vi "PythonIDE 3.vi"(7 "Python version":string="3.9", 9 "Processor":u16(ring) items=["SPIKE", "Pi"], 11 "Port":string) -> ()   [LabVIEW 2020]
uses:
  <vilib>/event_ctls.llb/eventvkey.ctl
  Serial_Global.vi
panel:
  out "Shift":bool
  in  "Explorer":u16(ring) items=["Explore...", "", "Arm", "Motors", "Scope", "Twin"]
  out "Buffer":i32(slide) scale=0.0..10000.0
  in  "Folder Path":path
  in  "Open PC":bool
  in  "reconnect":bool
  out "VKey":T1
  in  "Browser":bool
  in  "Tree":string(tree)
  in  "Spaces":bool
  in  "Name":string="main.py"
  in  "Save SPIKE":bool
  out "Script":string
  in  "Python Code":string
  out "Console":string
  in  "Clear":bool
  in  "Text.Font:Size":u32=12
  in  "Save Log":bool
  in  "Save PC":bool
  in  "stop":bool
  in  "Ctrl C":bool
  in  "run":bool
  # "PyVIEW IDE\nversion 0.1b10"
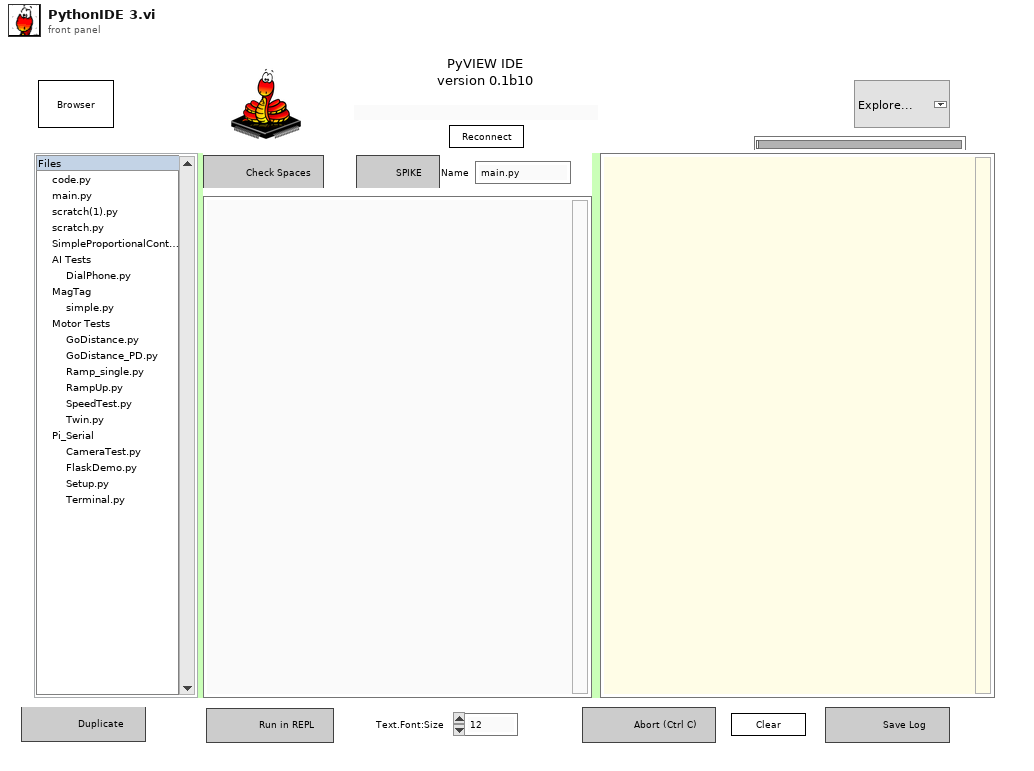
[diagram p1: front panel]
types:
  T1 = typedef "eventvkey.ctl" = enum16{"ASCII", "Enter", "Return", "Shift", "Ctrl", "Alt", "Cmd", "Opt", "Caps", "NumLock", "Clear", "Break", "Up", "Down", "Left", "Right", "Insert", "Delete", "Home", "End", "PageUp", "PageDown", "Escape", "Help", "Pause", "ScrollLock", "F1", "F2", "F3", "F4", "F5", "F6", "F7", "F8", "F9", "F10", "F11", "F12", "F13", "F14", "F15", "F16", "F17", "F18", "F19", "F20", "F21", "F22", "F23", "F24", "Play", "VolumeUp", "VolumeDown", "Mute", "Two Byte Char"}
  T2 = typedef "PythonCtrl.ctl" = cluster{"session":refnum<k35>, "PyPath":path, "Processor":enum16{"SPIKE", "Pi"}}
  T3 = enum8{"Enabled", "Disabled", "Disabled and Grayed Out"}
  T4 = typedef "Preferences.ctl" = cluster{"python":string, "arduino15":path, "arduino Lib":path, "pythonCode":path, "FontSize":u8}
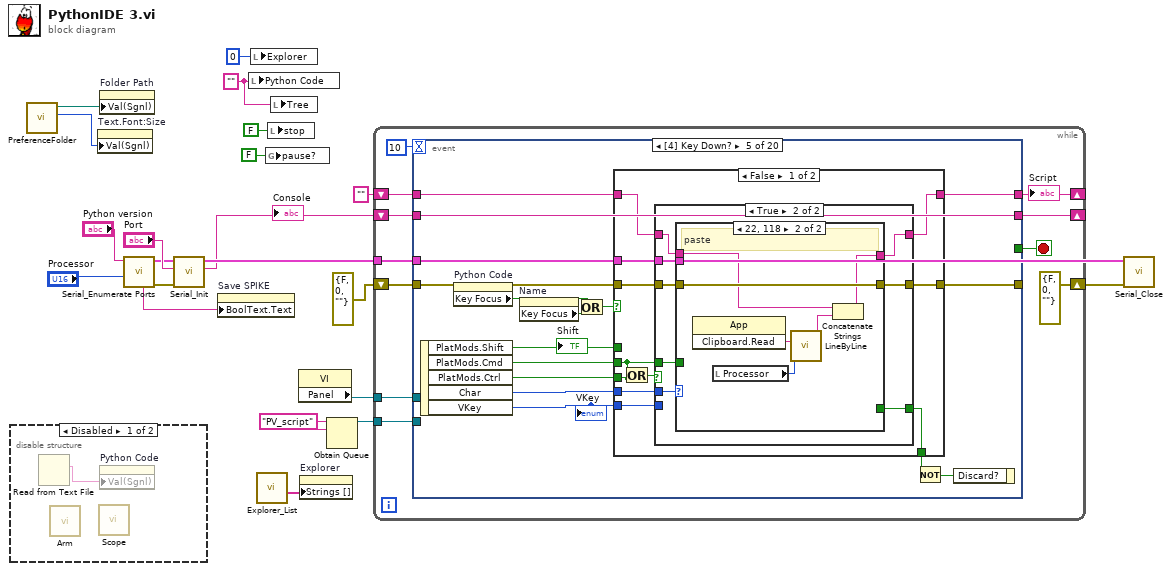
[diagram p0: block diagram]
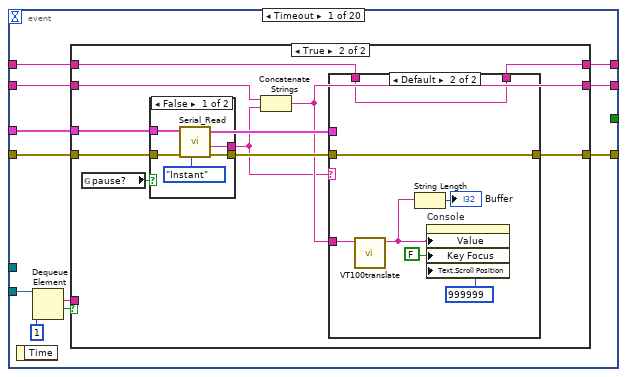
[diagram p2: hidden frame]
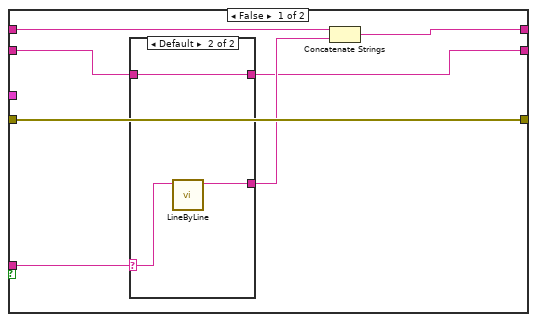
[diagram p3: hidden frame]
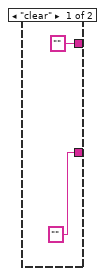
[diagram p4: hidden frame]
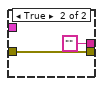
[diagram p5: hidden frame]
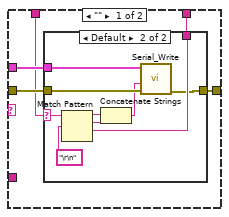
[diagram p6: hidden frame]
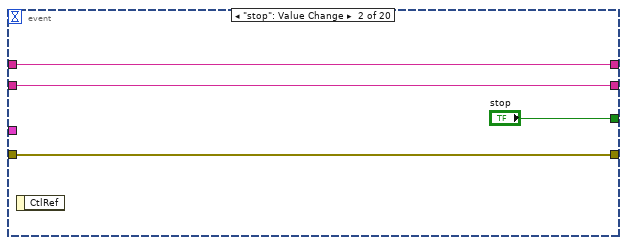
[diagram p8: hidden frame]
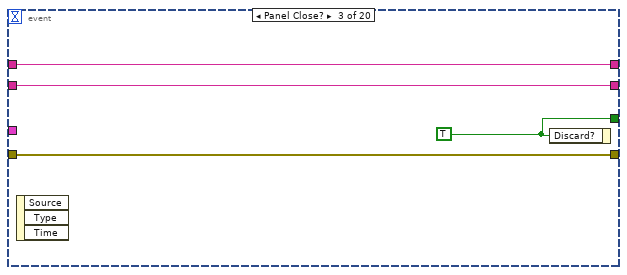
[diagram p9: hidden frame]
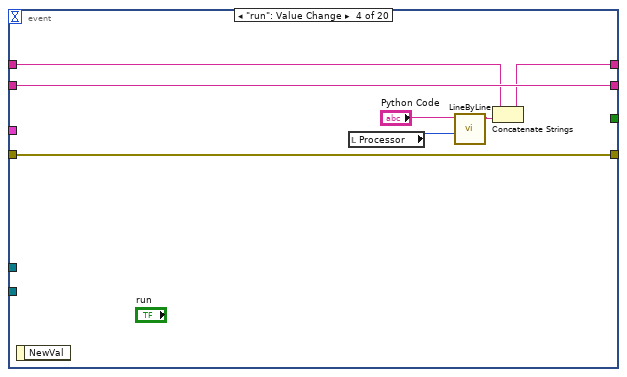
[diagram p10: hidden frame]
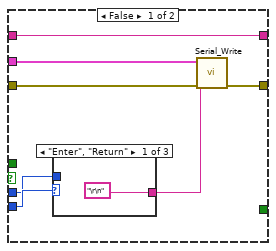
[diagram p11: hidden frame]
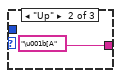
[diagram p12: hidden frame]
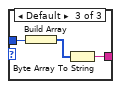
[diagram p13: hidden frame]
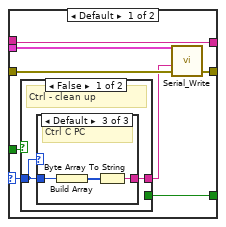
[diagram p14: hidden frame]
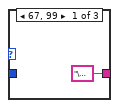
[diagram p15: hidden frame]
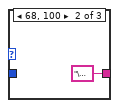
[diagram p16: hidden frame]
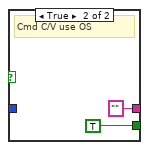
[diagram p17: hidden frame]
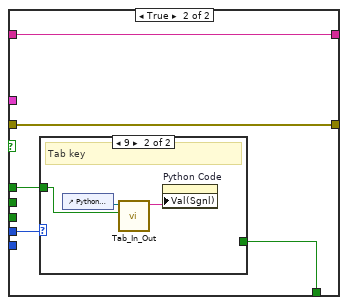
[diagram p18: hidden frame]
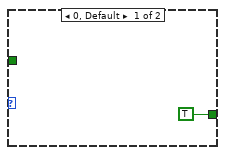
[diagram p19: hidden frame]
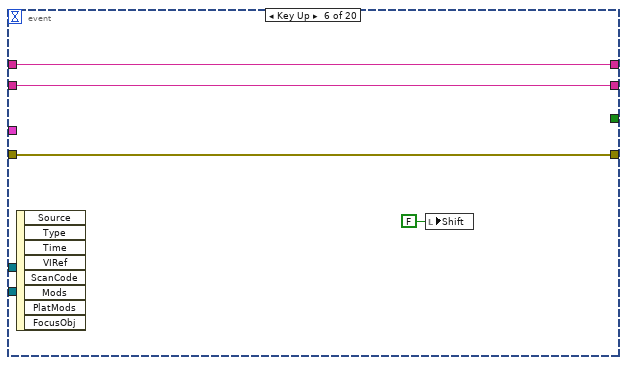
[diagram p20: hidden frame]
diagram:
  w6 = "PV_script" ("name (unnamed)")
  w11 = "" ("Python Code")
  n1 = disable-structure shown="Disabled" {
    frame Disabled {
      n2 = Read from Text File() -> (text=w22:string)  [unwired: 4 in, 3 out]
      n3 = call "Arm.vi"() -> ()  [unwired: 12 in]
      n4 = call "Scope.vi"() -> ()  [unwired: 12 in]
      n5 = property on="Python Code" class="Str"("Val(Sgnl)"=w22) -> ()  [unwired: 2 in, 2 out]
    }
    frame Enabled {
    }
  }
  n6 = call "PreferenceFolder.vi"() -> ("FontSize"=w9:u8, "pythonCode"=w10:path)  [unwired: 9 in, 1 out]
  n7 = property on="Text.Font:Size" class="DigNum (strict)"("Val(Sgnl)"=w9) -> ()  [unwired: 2 in, 2 out]
  n8 = property on="Folder Path" class="Path"("Val(Sgnl)"=w10) -> ()  [unwired: 2 in, 2 out]
  n9 = call "Serial_Enumerate Ports.vi"("Processor"="Processor", "Python version"="Python version") -> ("error out"=w15:errorcluster, "Python"=w17:T2, "name"=w1:string)  [unwired: 5 in, 2 out]
  n10 = call "Serial_Init.vi"("error in (no error)"=w15, "Port"="Port", "Python"=w17) -> ("Console"=w14:string, "Python out"=w16:T2)  [unwired: 6 in, 1 out]
  "Console" <- w14
  n11 = property on="Save SPIKE" class="Bool"("BoolText.Text"=w1) -> ()  [unwired: 2 in, 2 out]
  n12 = local write "Python Code"(w11) -> ()
  n13 = local write "Explorer"(0) -> ()
  n14 = call "Explorer_List.vi"() -> ("Options"=w3:string[])  [unwired: 9 in, 2 out]
  n15 = global write "Serial_Global.vi" "pause?"(FALSE ("pause?")) -> ()
  n16 = local write "stop"(FALSE ("stop")) -> ()
  n17 = local write "Tree"(w11) -> ()
  n18 = property class="VI"() -> ("Panel"=w18:refnum<vi>)  [unwired: 2 in, 2 out]
  n19 = property on="Explorer" class="Ring (strict)"("Strings []"=w3) -> ()  [unwired: 2 in, 2 out]
  n20 = Obtain Queue(name (unnamed)=w6, element data type=w6) -> (queue out=w5:refnum<queue>)  [unwired: 3 in, 2 out]
  n21 = while {
    shift-right: [w32] -> _
    shift-left: w14 -> [w33]
    shift-right: [errorcluster {"status"=FALSE, "code"=0, "source"=""} ("error IO")] -> w7
    shift-left: errorcluster {"status"=FALSE, "code"=0, "source"=""} ("error IO") -> [w29]
    tunnel: w18 -> [w28]
    shift-right: [w26] -> _
    shift-left: "" -> [w27]
    tunnel: w16 -> [w25]
    tunnel: w5 -> [w24]
    stop <- w31 stop-if-true
    n22 = event shown="[4] Key Down?" {
      selector: _ -> [_ _ _ _ _ _ _ _ _ _ _ _ _ _ _ _ _ _ _ _]
      dyn-events: _ -> [_ _ _ _ _ _ _ _ _ _ _ _ _ _ _ _ _ _ _ _]
      timeout: 10 -> [_ _ _ _ _ _ _ _ _ _ _ _ _ _ _ _ _ _ _ _]
      tunnel: w25 -> [w38 _ _ _ w127 _ w199 _ _ _ w245 _ _ _ w282 _ _ _ _ _]
      tunnel: w33 -> [w44 w99 w104 w111 w126 w193 w200 w210 w222 w236 w242 w252 w271 w276 w284 w297 w304 _ w316 w327]
      tunnel: [w43 w99 w104 w111 w126 w193 w200 w210 w222 w236 w242 w252 w271 w276 w284 w297 w304 w313 w316 w327] -> w32
      tunnel: [_ "stop" w101 _ _ _ _ _ _ _ _ _ _ _ _ _ _ _ _ _] -> w31
      tunnel: w29 -> [w39 w98 w103 w110 w120 w192 w198 w209 w221 w235 w244 w251 w272 w277 w281 w295 w302 w314 w321 w329]
      tunnel: [w42 w98 w103 w110 w121 w192 w196 w209 w221 w235 w243 w251 w272 w277 w278 w295 w302 w314 w321 w329] -> _
      tunnel: w28 -> [_ _ _ _ _ _ _ w208 w217 _ _ _ _ _ _ w292 _ _ _ _]
      tunnel: [w41 w97 w102 w108 w117 w194 "" w207 w223 w237 w246 w253 w270 w275 w283 w296 w303 w310 w320 w328] -> w26
      tunnel: w27 -> [w40 w97 w102 w109 w118 w194 _ w207 w223 w237 w246 w253 w270 w275 w283 w296 w303 w312 w320 w328]
      tunnel: w24 -> [w37 _ _ _ _ _ _ _ _ _ _ _ _ _ _ _ _ _ _ _]
      event Timeout {
        n23 = event-data() -> ()  [unwired: 1 in, 1 out]
        n24 = Dequeue Element(queue=w37, timeout in ms (-1)=1) -> (element=w34:string, timed out?=w35:bool)  [unwired: 1 in, 2 out]
        n25 = case shown="True" w35 {
          tunnel: w44 -> [w45 w66]
          tunnel: [w46 w58] -> w43
          tunnel: [w51 w65] -> w42
          tunnel: [w49 w64] -> w41
          tunnel: w40 -> [w50 w63]
          tunnel: w39 -> [w51 w62]
          tunnel: w38 -> [_ w60]
          tunnel: w34 -> [w47 _]
          frame False {
            n26 = case shown="Default" w47 {
              selector: w47 -> [_ w54]
              tunnel: ["" ("result string") w56] -> w48
              tunnel: ["" ("Console") w55] -> w46
              tunnel: w45 -> [_ w55]
              frame "clear" {
              }
              frame Default {
                n27 = call "LineByLine.vi"("Python Code"=w54) -> ("result string"=w56:string)  [unwired: 10 in]
              }
            }
            n28 = Concatenate Strings(w50, w48) -> (w49:string)
          }
          frame True {
            n29 = global read "Serial_Global.vi" "pause?"() -> (w59:bool)
            n30 = case shown="False" w59 {
              tunnel: w62 -> [w71 w73]
              tunnel: [w70 "" ("Text read")] -> w57
              tunnel: [w69 w73] -> w61
              tunnel: w60 -> [w68 _]
              frame False {
                n31 = call "Serial_Read.vi"("Task"=enum16{"Instant", "All"}."Instant", "error in (no error)"=w71, "Python"=w68) -> ("error out"=w69:errorcluster, "Text read"=w70:string)  [unwired: 7 in]
              }
              frame True {
              }
            }
            n32 = Concatenate Strings(w66, w57) -> (w58:string)
            n33 = case shown="Default" w57 {
              tunnel: w58 -> [_ w96]
              tunnel: w61 -> [w77 w93]
              tunnel: [w76 w93] -> w65
              tunnel: w63 -> [w74 w92]
              tunnel: [w78 w92] -> w64
              tunnel: w60 -> [w75 _]
              frame "" {
                n34 = case shown="Default" w74 {
                  selector: w74 -> [w80 w81]
                  tunnel: [w80 w89] -> w78
                  tunnel: w77 -> [w79 w85]
                  tunnel: [w79 w84] -> w76
                  tunnel: w75 -> [_ w82]
                  frame "" {
                  }
                  frame Default {
                    n35 = Match Pattern(string=w81, regular expression="\r\n") -> (before substring=w87:string, match substring=w86:string, after substring=w89:string)  [unwired: 1 in, 1 out]
                    n36 = Concatenate Strings(w87, w86) -> (w83:string)
                    n37 = call "Serial_Write.vi"("error in (no error)"=w85, "Text to write"=w83, "Python"=w82) -> ("error out"=w84:errorcluster)  [unwired: 8 in]
                  }
                }
              }
              frame Default {
                n38 = call "VT100translate.vi"("Console"=w96) -> ("Console 2"=w90:string)  [unwired: 10 in]
                n39 = String Length(string=w90) -> (length=→"Buffer":i32)
                n40 = property on="Console" class="Str"("Value"=w90, "Key Focus"=FALSE, "Text.Scroll Position"=u32 999999) -> ()  [unwired: 2 in, 2 out]
              }
            }
          }
        }
      }
      event "stop": Value Change {
        n41 = event-data() -> ()  [unwired: 1 in, 1 out]
      }
      event Panel Close? {
        w101 = TRUE ("stop")
        n42 = event-data() -> ()  [unwired: 1 in, 3 out]
        n43 = event-data("Discard?"=w101) -> ()  [unwired: 1 in, 1 out]
      }
      event "run": Value Change {
        n44 = event-data() -> ()  [unwired: 1 in, 1 out]
        n45 = local read "Processor"() -> (w105:u16)
        n46 = call "LineByLine.vi"("Processor"=w105, "Python Code"="Python Code") -> ("result string"=w107:string)  [unwired: 9 in]
        n47 = Concatenate Strings(w109, w107) -> (w108:string)
      }
      event Key Down? {
        n48 = event-data() -> ("PlatMods.Shift"=w112:bool, "PlatMods.Cmd"=w122:bool, "PlatMods.Ctrl"=w123:bool, "Char"=w124:i16, "VKey"=w125:T1)  [unwired: 1 in]
        "VKey" <- w125
        "Shift" <- w112
        n49 = property on="Python Code" class="Str"() -> ("Key Focus"=w114:bool)  [unwired: 2 in, 2 out]
        n50 = property on="Name" class="Str"() -> ("Key Focus"=w115:bool)  [unwired: 2 in, 2 out]
        n51 = Or(x=w114, y=w115) -> (x .or. y?=w113:bool)
        n52 = case shown="False" w113 {
          tunnel: w127 -> [w136 _]
          tunnel: w125 -> [w138 _]
          tunnel: w124 -> [w137 w184]
          tunnel: w123 -> [w129 _]
          tunnel: w122 -> [w130 _]
          tunnel: [w134 w186] -> w121
          tunnel: w120 -> [w135 w186]
          tunnel: [w131 w183] -> w119
          tunnel: w118 -> [w133 w185]
          tunnel: [w132 w185] -> w117
          tunnel: w112 -> [_ w182]
          frame False {
            n53 = Or(x=w130, y=w129) -> (x .or. y?=w128:bool)
            n54 = case shown="True" w128 {
              tunnel: w138 -> [w145 _]
              tunnel: w137 -> [w144 w158]
              tunnel: w136 -> [w143 w157]
              tunnel: w135 -> [w142 w156]
              tunnel: [w140 w155] -> w134
              tunnel: w133 -> [w139 w154]
              tunnel: [w139 w153] -> w132
              tunnel: w130 -> [_ w152]
              tunnel: [_ w151] -> w131
              frame False {
                n55 = case shown="\"Enter\", \"Return\"" w145 {
                  tunnel: w144 -> [_ _ w150]
                  tunnel: ["\r\n" ("replace string (\"\")") "\u001b[A" ("replace string (\"\")") w148] -> w141
                  frame "Enter", "Return" {
                  }
                  frame "Up" {
                  }
                  frame Default {
                    n56 = Build Array(w150) -> (w149:i16[])
                    n57 = Byte Array To String(unsigned byte array=w149) -> (string=w148:string)
                  }
                }
                n58 = call "Serial_Write.vi"("error in (no error)"=w142, "Text to write"=w141, "Python"=w143) -> ("error out"=w140:errorcluster)  [unwired: 8 in]
              }
              frame True {
                n59 = case shown="22, 118" w158 {
                  selector: w158 -> [w161 _]
                  tunnel: w157 -> [w166 _]
                  tunnel: w156 -> [w165 w181]
                  tunnel: [w164 w181] -> w155
                  tunnel: w154 -> [w162 w180]
                  tunnel: [w162 w179] -> w153
                  tunnel: w152 -> [w160 _]
                  tunnel: [w159 _] -> w151
                  frame Default {
                    n60 = case shown="False" w160 {
                      tunnel: [w168 "" ("string")] -> w163
                      tunnel: w161 -> [w167 _]
                      tunnel: [_ TRUE ("Discard?")] -> w159
                      frame False {
                        # "Ctrl - clean up"
                        n61 = case shown="Default" w167 {
                          tunnel: w167 -> [_ _ w172]
                          tunnel: ["\u0003" ("string") "\u0004" ("string") w171] -> w168
                          frame 67, 99 {
                          }
                          frame 68, 100 {
                          }
                          frame Default {
                            # "Ctrl C PC"
                            n62 = Build Array(w172) -> (w173:i16[])
                            n63 = Byte Array To String(unsigned byte array=w173) -> (string=w171:string)
                          }
                        }
                      }
                      frame True {
                        # "Cmd C/V use OS"
                      }
                    }
                    n64 = call "Serial_Write.vi"("error in (no error)"=w165, "Text to write"=w163, "Python"=w166) -> ("error out"=w164:errorcluster)  [unwired: 8 in]
                  }
                  frame 22, 118 {
                    # "paste"
                    n65 = invoke class="App" method="Clipboard.Read"() -> ("Read Clipbrd"=w178:string)  [unwired: 3 in, 2 out]
                    n66 = local read "Processor"() -> (w176:u16)
                    n67 = call "LineByLine.vi"("Processor"=w176, "Python Code"=w178) -> ("result string"=w177:string)  [unwired: 9 in]
                    n68 = Concatenate Strings(w180, w177) -> (w179:string)
                  }
                }
              }
            }
          }
          frame True {
            n69 = case shown="9" w184 {
              tunnel: [TRUE ("Discard?") _] -> w183
              tunnel: w182 -> [_ w189]
              frame 0, Default {
              }
              frame 9 {
                # "Tab key"
                n70 = control-ref of="Python Code"() -> (w190:refnum<vi>)
                n71 = call "Tab_In_Out.vi"("Shift?"=w189, "String in"=w190) -> ("result string"=w188:string)  [unwired: 9 in]
                n72 = property on="Python Code" class="Str"("Val(Sgnl)"=w188) -> ()  [unwired: 2 in, 2 out]
              }
            }
          }
        }
        n73 = Not(x=w119) -> (.not. x?=w116:bool)
        n74 = event-data("Discard?"=w116) -> ()  [unwired: 1 in, 1 out]
      }
      event Key Up {
        n75 = event-data() -> ()  [unwired: 1 in, 8 out]
        n76 = local write "Shift"(FALSE ("Shift")) -> ()
      }
      event "Ctrl C": Value Change {
        n77 = event-data() -> ()  [unwired: 1 in, 1 out]
        n78 = call "Serial_Write.vi"("error in (no error)"=w198, "Text to write"="\u0003\r\n\r\n" ("function name"), "Python"=w199) -> ("error out"=w196:errorcluster)  [unwired: 8 in]
      }
      event "Python Code": Value Change {
        n79 = event-data() -> ()  [unwired: 1 in, 1 out]
        n80 = local read "VKey"() -> (w205:T1)
        n81 = case shown="\"Enter\", \"Return\"" w205 {
          tunnel: [FALSE TRUE] -> w204
          frame Default {
          }
          frame "Enter", "Return" {
          }
        }
        n82 = control-ref of="Python Code"() -> (w206:refnum<vi>)
        n83 = call "Color_Assign.vi"("Add Spaces?"=w204, "Front Panel"=w208, "Code"=w206) -> ("Value"=w203:string)  [unwired: 8 in]
        n84 = property on="Python Code" class="Str"() -> ("DisabledEnum"=w201:T3)  [unwired: 2 in, 2 out]
        n85 = local read "Tree"() -> (w202:string)
        n86 = case shown="\"Enabled\"" w201 {
          tunnel: w203 -> [_ w213]
          tunnel: w202 -> [_ w212]
          frame Default {
          }
          frame "Enabled" {
            n87 = String To Path(string=w212) -> (path=w211:path)
            n88 = Write to Text File(file (use dialog)=w211, text=w213) -> ()  [unwired: 2 in, 3 out]
          }
        }
      }
      event "Save PC": Value Change {
        n89 = event-data() -> ()  [unwired: 1 in, 3 out]
        n90 = local read "Folder Path"() -> (w216:path)
        n91 = call "File Dialog"("start path"=w216, "default name"="Name") -> ("selected path"=w219:path, "error out"=w218:errorcluster)  [unwired: 10 in, 2 out]
        n92 = case shown="No Error" w218 {
          tunnel: w219 -> [w225 _]
          tunnel: w217 -> [w231 _]
          tunnel: w216 -> [w227 _]
          frame No Error {
            n93 = call "CheckForExtension.vi"("selected path"=w225) -> ("dup file"=w224:path)  [unwired: 10 in]
            n94 = local read "Python Code"() -> (w226:string)
            n95 = control-ref of="Tree"() -> (w230:refnum<vi>)
            n96 = Path To String(path=w224) -> (string=w228:string)
            n97 = Write to Text File(file (use dialog)=w224, text=w226) -> (error out=w229:errorcluster)  [unwired: 2 in, 2 out]
            n98 = call "InitializeTree.vi"("Folder path"=w227, "error in (no error)"=w229, "File"=w228, "Panel"=w231, "TreeControl in"=w230) -> ()  [unwired: 7 in]
          }
          frame Error {
          }
        }
      }
      event "Open PC": Value Change {
        n99 = event-data() -> ()  [unwired: 1 in, 3 out]
        n100 = local read "Folder Path"() -> (w232:path)
        n101 = call "File Dialog2"("start path"=w232) -> ("selected path"=w234:path, "error out"=w233:errorcluster)  [unwired: 11 in, 2 out]
        n102 = case shown="No Error" w233 {
          tunnel: w234 -> [w239 _]
          frame No Error {
            n103 = Read from Text File(file (use dialog)=w239) -> (text=w238:string)  [unwired: 3 in, 3 out]
            n104 = property on="Python Code" class="Str"("Val(Sgnl)"=w238) -> ()  [unwired: 2 in, 2 out]
          }
          frame Error {
          }
        }
      }
      event "Save SPIKE": Value Change {
        n105 = event-data() -> ()  [unwired: 1 in, 3 out]
        n106 = local read "Python Code"() -> (w240:string)
        n107 = local read "Name"() -> (w241:string)
        n108 = call "ReadFileDialog.vi"("File Text"=w240, "error in (no error)"=w244, "File name"=w241, "Python in"=w245) -> ("error out"=w243:errorcluster)  [unwired: 6 in, 1 out]
      }
      event "Explorer": Value Change {
        n109 = event-data() -> ("NewVal"=w248:u16)  [unwired: 1 in, 1 out]
        n110 = property on="Explorer" class="Ring (strict)"() -> ("Strings []"=w249:string[])  [unwired: 2 in, 2 out]
        n111 = Index Array(array=w249, index=w248) -> (element=w247:string)
        n112 = case shown="Default" w248 {
          tunnel: w247 -> [_ w258]
          frame 0 {
          }
          frame Default {
            n113 = local read "Shift"() -> (w257:bool)
            n114 = Select(t=enum16{"run", "open"}."open" ("Task"), s=w257, f=enum16{"run", "open"}."run" ("Task")) -> (s? t:f=w254:enum16{"run", "open"})
            n115 = control-ref of="Console"() -> (w259:refnum<vi>)
            n116 = call "Explore_Open.vi"("Task"=w254, "Name"=w258, "String in"=w259) -> ()  [unwired: 9 in]
          }
        }
        n117 = local write "Explorer"(0) -> ()
      }
      event "Browser": Value Change {
        w268 = 128  # call and forget
        n118 = event-data() -> ()  [unwired: 1 in, 3 out]
        n119 = vi-ref "Examples.vi"() -> (w265:refnum<vi>)
        n120 = property class="VI"(reference=w265) -> ("Name"=w266:string)  [unwired: 1 in, 2 out]
        n121 = local read "Port"() -> (w264:string)
        n122 = Open VI Reference(type specifier VI Refnum (for type only)=refnum<vi> refnum, vi path=w266, options=w268) -> (vi reference=w269:refnum<vi>, error out=w260:errorcluster)  [unwired: 3 in]
        n123 = local read "Python version"() -> (w263:string)
        n124 = call-by-ref "Start Asynchronous Call"(reference=w269, error in=w260, "Python version"=w263, "Port"=w264) -> (reference out=w261:refnum<vi>, error out=w262:errorcluster)  [unwired: 10 in]
        n125 = Close Reference(reference=w261, error in (no error)=w262) -> ()  [unwired: 1 out]
      }
      event "Spaces": Value Change {
        n126 = event-data() -> ()  [unwired: 1 in, 3 out]
        n127 = property on="Python Code" class="Str"() -> ("Value"=w273:string)  [unwired: 2 in, 2 out]
        n128 = call "CleanUp.vi"("Python Code"=w273) -> ("spreadsheet string"=w274:string)  [unwired: 10 in]
        n129 = property on="Python Code" class="Str"("Val(Sgnl)"=w274) -> ()  [unwired: 2 in, 2 out]
      }
      event "reconnect": Value Change {
        n130 = event-data() -> ()  [unwired: 1 in, 3 out]
        n131 = flat-sequence {
          tunnel: w282 -> [w285]
          tunnel: w281 -> [w286]
          tunnel: [w285] -> w279
          tunnel: [w287] -> w280
          tunnel: w279 -> [w287]
          tunnel: w280 -> [w290]
          tunnel: [w288] -> w278
          frame #0 {
            n132 = call "Serial_Close.vi"("error in (no error)"=w286, "Python in"=w285) -> ()  [unwired: 10 in]
          }
          frame #1 {
          }
          frame #2 {
            n133 = local read "Port"() -> (w289:string)
            n134 = call "Serial_Init.vi"("Port"=w289, "Python"=w290) -> ("error out"=w288:errorcluster)  [unwired: 7 in, 2 out]
          }
        }
      }
      event "Folder Path": Value Change {
        # "Reset path to Code Folder"
        n135 = event-data() -> ()  [unwired: 1 in, 3 out]
        n136 = control-ref of="Tree"() -> (w294:refnum<vi>)
        n137 = call "InitializeTree.vi"("Folder path"="Folder Path", "File"="scratch.py" ("Python Code"), "Panel"=w292, "TreeControl in"=w294) -> ()  [unwired: 8 in]
      }
      event "Tree": Value Change {
        # "rebuild tree and load new file"
        n138 = event-data() -> ()  [unwired: 1 in, 3 out]
        n139 = String To Path(string="Tree") -> (path=w299:path)
        n140 = Read from Text File(file (use dialog)=w299) -> (text=w300:string, error out=w298:errorcluster)  [unwired: 3 in, 2 out]
        n141 = case shown="No Error" w298 {
          tunnel: w300 -> [w306 _]
          frame No Error {
            n142 = property on="Python Code" class="Str"("Val(Sgnl)"=w306, "DisabledEnum"=T3."Enabled" ("Disabled")) -> ()  [unwired: 2 in, 2 out]
          }
          frame Error {
            n143 = property on="Python Code" class="Str"("Val(Sgnl)"="" ("Python Code"), "DisabledEnum"=T3."Disabled and Grayed Out" ("Disabled")) -> ()  [unwired: 2 in, 2 out]
          }
        }
      }
      event "Clear": Value Change {
        w313 = ""
        n144 = event-data() -> ()  [unwired: 1 in, 3 out]
        n145 = Concatenate Strings(w312, "\r\n" ("string")) -> (w310:string)
        n146 = local write "Console"(w313) -> ()
        n147 = local write "Buffer"(0) -> ()
      }
      event "Save Log": Value Change {
        n148 = event-data() -> ()  [unwired: 1 in, 3 out]
        n149 = local read "Folder Path"() -> (w318:path)
        n150 = call "File Dialog3"("start path"=w318, "default name"="log.txt") -> ("selected path"=w315:path, "error out"=w317:errorcluster)  [unwired: 10 in, 2 out]
        n151 = case shown="No Error" w317 {
          tunnel: w316 -> [w323 _]
          tunnel: w315 -> [w322 _]
          frame No Error {
            n152 = Write to Text File(file (use dialog)=w322, text=w323) -> ()  [unwired: 2 in, 3 out]
          }
          frame Error {
          }
        }
      }
      event "Text.Font:Size": Value Change {
        n153 = event-data() -> ()  [unwired: 1 in, 3 out]
        n154 = call "Preferences.vi"() -> ("Preferences out"=w324:T4)  [unwired: 10 in, 1 out]
        n155 = Bundle By Name(cluster=w324, "FontSize"="Text.Font:Size") -> (w326:T4)
        n156 = property on="Python Code" class="Str"("Text.FontSize"="Text.Font:Size") -> ()  [unwired: 2 in, 2 out]
        n157 = call "Preferences.vi"("Preferences in"=w326) -> ()  [unwired: 9 in, 2 out]
      }
    }
    "Script" <- w26
  }
  n158 = call "Serial_Close.vi"("error in (no error)"=w7, "Python in"=w16) -> ()  [unwired: 10 in]
